vi "magnet_ps_pd_read.vi"(8 "error in (no error)":errorcluster, 10 "byte count to read":u32=12, 11 "VISA resource name":refnum<visa-resource-name>) -> (0 "error out":errorcluster, 1 "Shim Coil 2":bool, 2 "Shim Coil 1":bool, 3 "VISA resource name out":refnum<visa-resource-name>, 4 "Background intensity (raw)":i32, 5 "read buffer":string, 6 "High Background?":bool)   [LabVIEW 2019]
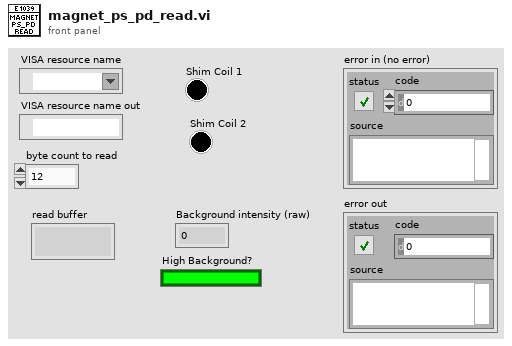
[diagram p1: front panel]
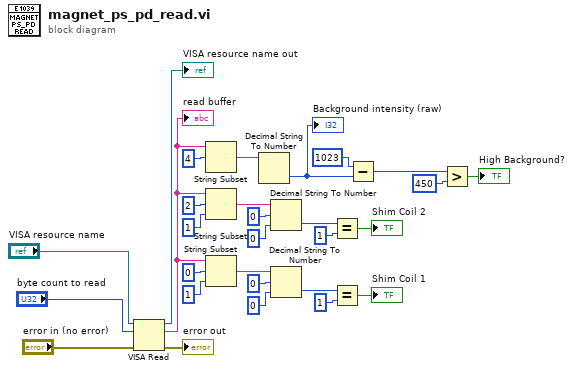
[diagram p0: block diagram]
diagram:
  n1 = VISA Read(VISA resource name="VISA resource name", byte count="byte count to read", error in (no error)="error in (no error)") -> (VISA resource name out=→"VISA resource name out":refnum<visa-resource-name>, read buffer=w13:string, error out=→"error out":errorcluster)  [unwired: 1 out]
  "read buffer" <- w13
  n2 = String Subset(string=w13, offset (0)=4) -> (substring=w11:string)  [unwired: 1 in]
  n3 = String Subset(string=w13, offset (0)=2, length (rest)=1 ("length (rest)")) -> (substring=w19:string)
  n4 = String Subset(string=w13, offset (0)=0, length (rest)=1 ("length (rest)")) -> (substring=w25:string)
  n5 = Decimal String To Number(string=w11) -> (number=w3:i32)  [unwired: 2 in, 1 out]
  "Background intensity (raw)" <- w3
  n6 = Decimal String To Number(string=w19, offset=0, default (0L)=0 ("default (0 I32)")) -> (number=w16:i32)  [unwired: 1 out]
  n7 = Decimal String To Number(string=w25, offset=0, default (0L)=0 ("default (0 I32)")) -> (number=w22:i32)  [unwired: 1 out]
  n8 = Equal?(x=w16, y=1) -> (x = y?=→"Shim Coil 2":bool)
  n9 = Equal?(x=w22, y=1) -> (x = y?=→"Shim Coil 1":bool)
  n10 = Subtract(x=1023, y=w3) -> (x-y=w1:i32)
  n11 = Greater?(x=w1, y=450) -> (0:→"High Background?":bool)
